vi "Scale pDataBuffer.vi"(5 "Min":u16, 7 "Max":u16, 10 "pDataBuffer":u16[](array[numeric])) -> (2 "Scaled pDataBuffer":u16[](array[numeric]))   [LabVIEW 2020]
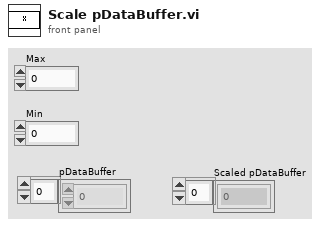
[diagram p1: front panel]
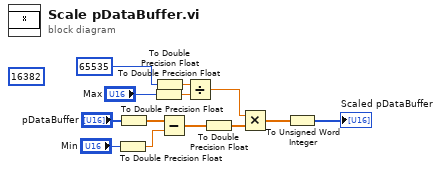
[diagram p0: block diagram]
diagram:
  (unwired) u16 16382
  n1 = To Double Precision Float(number="Min") -> (double precision float=w2:dbl)
  n2 = To Double Precision Float(number="pDataBuffer") -> (double precision float=w3:dbl[])
  n3 = To Double Precision Float(number="Max") -> (double precision float=w10:dbl)
  n4 = To Double Precision Float(number=u16 65535) -> (double precision float=w12:dbl)
  n5 = Subtract(x=w3, y=w2) -> (x-y=w9:dbl[])
  n6 = Divide(x=w12, y=w10) -> (x/y=w8:dbl)
  n7 = To Double Precision Float(number=w9) -> (double precision float=w7:dbl[])
  n8 = Multiply(x=w8, y=w7) -> (x*y=w6:dbl[])
  n9 = To Unsigned Word Integer(number=w6) -> (unsigned 16bit integer=→"Scaled pDataBuffer":u16[])
